vi "FIx thing.vi"(1 "Input":T1) -> (0 "Output":T1)   [LabVIEW 2018]
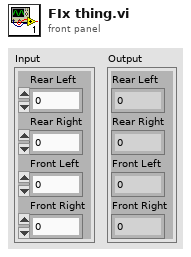
[diagram p1: front panel]
types:
  T1 = cluster{"Rear Left":dbl, "Rear Right":dbl, "Front Left":dbl, "Front Right":dbl}
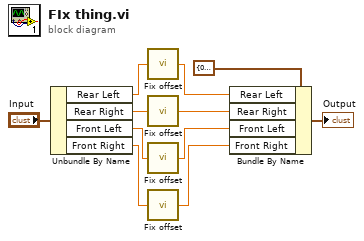
[diagram p0: block diagram]
diagram:
  n1 = Unbundle By Name("Input") -> ("Rear Left"=w10:dbl, "Rear Right"=w9:dbl, "Front Left"=w8:dbl, "Front Right"=w7:dbl)
  n2 = call "Fix offset.vi"("Input"=w10) -> ("Output"=w5:dbl)
  n3 = call "Fix offset.vi"("Input"=w9) -> ("Output"=w4:dbl)
  n4 = call "Fix offset.vi"("Input"=w8) -> ("Output"=w3:dbl)
  n5 = call "Fix offset.vi"("Input"=w7) -> ("Output"=w2:dbl)
  n6 = Bundle By Name(cluster=T1 {"Rear Left"=0.0, "Rear Right"=0.0, "Front Left"=0.0, "Front Right"=0.0} ("Output 2"), "Rear Left"=w5, "Rear Right"=w4, "Front Left"=w3, "Front Right"=w2) -> (→"Output":T1)
